vi "Write Connected Msg.vi"(10 "Connected Msg":refnum<class "Connected Msg.lvclass">, 11 "Legacy Nested Endpoint in":refnum<class "Legacy Nested Endpoint.lvclass">) -> (3 "Legacy Nested Endpoint out":refnum<class "Legacy Nested Endpoint.lvclass">)   [LabVIEW 2020, in "Legacy Nested Endpoint.lvlib" / "Legacy Nested Endpoint.lvclass"]
doc: "Use this VI to specify the message type to be sent to this actor's caller after a connection has been established. The type must be a child of the Connected Msg class.\n\nYou must specify this message class prior to launching the actor."
uses:
  <vilib>/NI/Actors/Network Endpoint Actors/Legacy Nested Endpoint/Legacy Nested Endpoint/Legacy Nested Endpoint.lvclass
  <vilib>/NI/Actors/Network Endpoint Actors/Legacy Nested Endpoint/Legacy Nested Endpoint Messages/Connected Msg/Connected Msg.lvclass
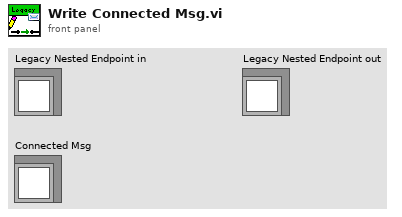
[diagram p1: front panel]
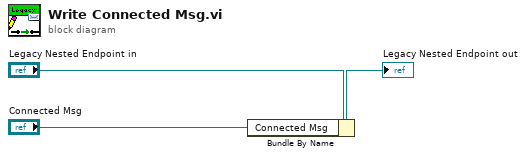
[diagram p0: block diagram]
diagram:
  n1 = Bundle By Name(cluster="Legacy Nested Endpoint in", "Connected Msg"="Connected Msg") -> (→"Legacy Nested Endpoint out":refnum<class "Legacy Nested Endpoint.lvclass">)
